vi "SMOOTHIE MAIN.vi"() -> ()   [LabVIEW 2016]
uses:
  PROCESSES.ctl
  <vilib>/Instr/_visa.llb/VISA Open Access Mode.ctl
panel:
  out "elements":T1[](array[typedef])
  out "CONNECTED":bool
  in  "ENABLE XYZ":bool
  out "GOTO STRING":string
  in  "ABS":bool
  in  "GOTO POSITION":T2 {"Z" format="%_4g"; "Y" min=-0.019999999552965164 max=0.019999999552965164 step=9.999999747378752e-05 format="%_5g"; "X" format="%_5g"}
  out "APOS":string
  in  "Stop Button":bool
  out "LIMITS":string
  in  "LIMITS":bool
  out "SMOOTHIE VISA":refnum<visa-resource-name>
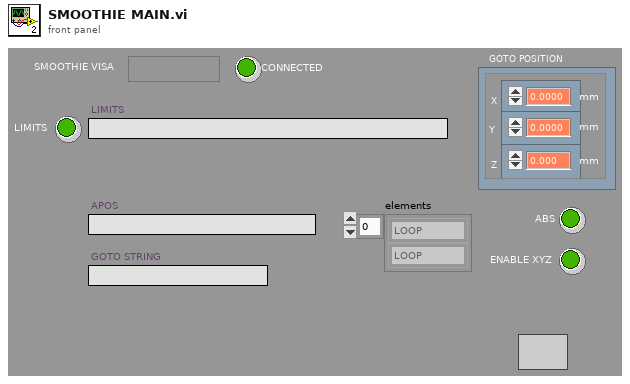
[diagram p1: front panel]
types:
  T1 = typedef "PROCESSES.ctl" = enum16{"LOOP", "LIMITS SETTINGS", "INITIALISE COMM", "CLOSE VISA COMM", "ACTUATOR POSITIONS", "GOTO POSITION (TOOL UP)", "ABSOLUTE or RELATIVE", "ENABLE STEPPER MOTORS"}
  T2 = cluster{"X":dbl[unit], "Y":dbl[unit], "Z":dbl[unit]}
  T3 = typedef "VISA Open Access Mode.ctl" = u32
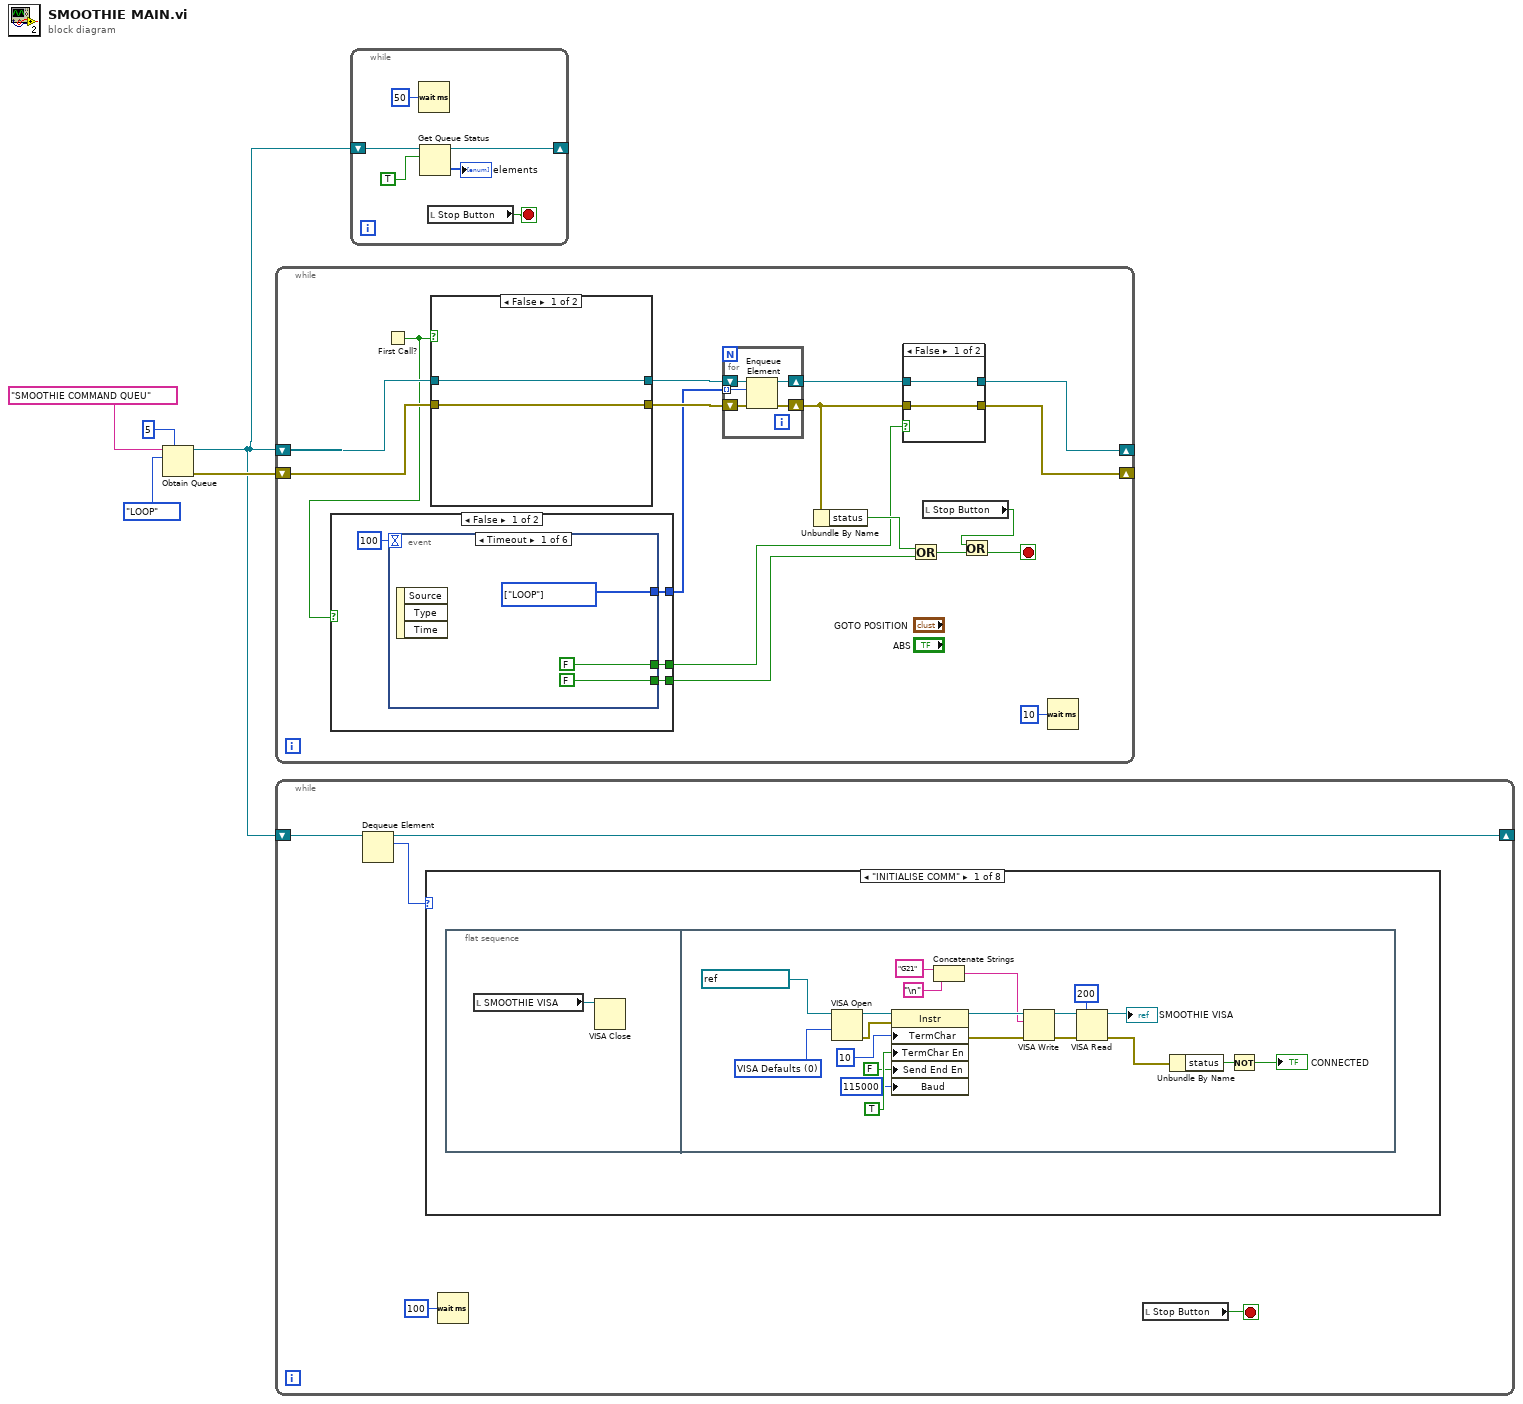
[diagram p0: block diagram]
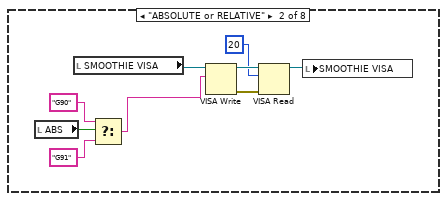
[diagram p2: hidden frame]
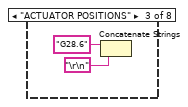
[diagram p3: hidden frame]
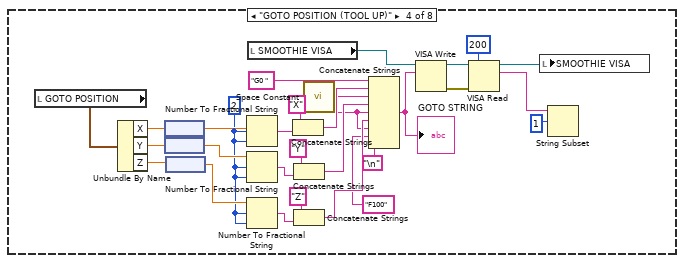
[diagram p4: hidden frame]
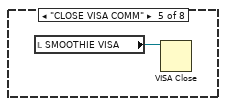
[diagram p5: hidden frame]
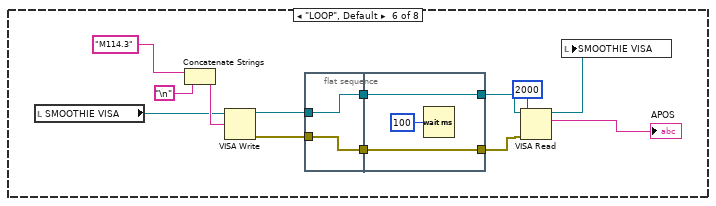
[diagram p6: hidden frame]
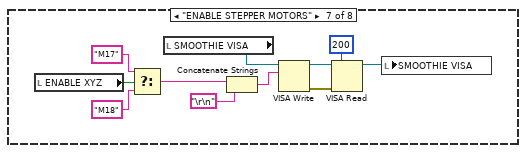
[diagram p7: hidden frame]
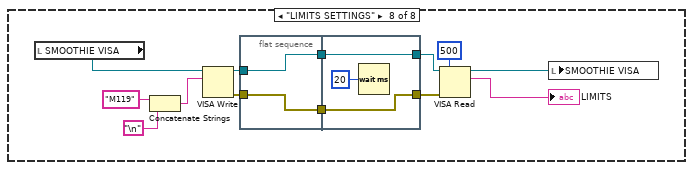
[diagram p8: hidden frame]
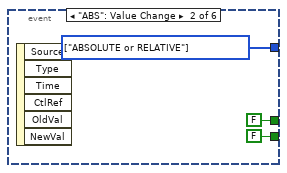
[diagram p9: hidden frame]
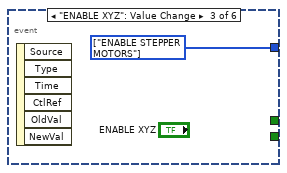
[diagram p10: hidden frame]
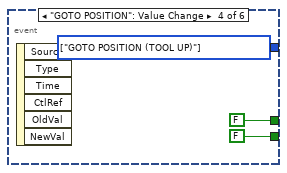
[diagram p11: hidden frame]
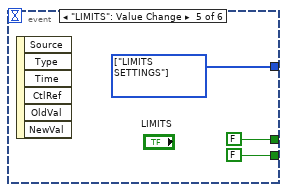
[diagram p12: hidden frame]
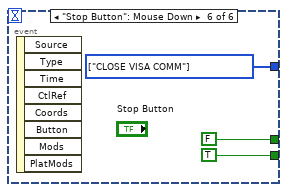
[diagram p13: hidden frame]
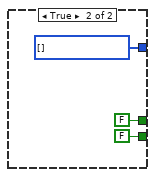
[diagram p14: hidden frame]
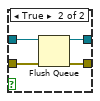
[diagram p15: hidden frame]
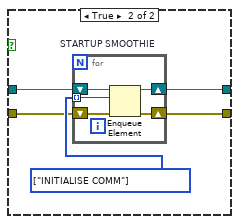
[diagram p16: hidden frame]
diagram:
  n1 = Obtain Queue(max queue size (-1, unlimited)=5, name (unnamed)="SMOOTHIE COMMAND QUEU", element data type=PROCESSES."LOOP") -> (queue out=w1:refnum<queue>, error out=w4:errorcluster)  [unwired: 2 in, 1 out]
  n2 = while {
    shift-right: [w11] -> _
    shift-left: w1 -> [w22]
    shift-right: [w10] -> _
    shift-left: w4 -> [w21]
    stop <- w9 stop-if-true
    n3 = First Call?() -> (First Call?: T/F=w12:bool)
    n4 = case shown="False" w12 {
      tunnel: [w25 w45] -> w18
      tunnel: [w24 FALSE] -> w16
      tunnel: [w23 FALSE] -> w14
      frame False {
        n5 = event shown="[0] Timeout" {
          selector: _ -> [_ _ _ _ _ _]
          dyn-events: _ -> [_ _ _ _ _ _]
          timeout: 100 -> [_ _ _ _ _ _]
          tunnel: [w29 w32 w33 w36 w39 w40] -> w25
          tunnel: [FALSE FALSE _ FALSE FALSE FALSE] -> w23
          tunnel: [FALSE FALSE _ FALSE FALSE TRUE] -> w24
          event Timeout {
            w29 = T1[] [enum."LOOP"] items=["LOOP", "LIMITS SETTINGS", "INITIALISE COMM", "CLOSE VISA COMM", "ACTUATOR POSITIONS", "GOTO POSITION (TOOL UP)", "ABSOLUTE or RELATIVE", "ENABLE STEPPER MOTORS"]
            n6 = event-data() -> ()  [unwired: 1 in, 3 out]
          }
          event "ABS": Value Change {
            w32 = T1[] [enum."ABSOLUTE or RELATIVE"] items=["LOOP", "LIMITS SETTINGS", "INITIALISE COMM", "CLOSE VISA COMM", "ACTUATOR POSITIONS", "GOTO POSITION (TOOL UP)", "ABSOLUTE or RELATIVE", "ENABLE STEPPER MOTORS"]
            n7 = event-data() -> ()  [unwired: 1 in, 6 out]
          }
          event "ENABLE XYZ": Value Change {
            w33 = T1[] [enum."ENABLE STEPPER MOTORS"] items=["LOOP", "LIMITS SETTINGS", "INITIALISE COMM", "CLOSE VISA COMM", "ACTUATOR POSITIONS", "GOTO POSITION (TOOL UP)", "ABSOLUTE or RELATIVE", "ENABLE STEPPER MOTORS"]
            n8 = event-data() -> ()  [unwired: 1 in, 6 out]
          }
          event "GOTO POSITION": Value Change {
            w36 = T1[] [enum."GOTO POSITION (TOOL UP)"] items=["LOOP", "LIMITS SETTINGS", "INITIALISE COMM", "CLOSE VISA COMM", "ACTUATOR POSITIONS", "GOTO POSITION (TOOL UP)", "ABSOLUTE or RELATIVE", "ENABLE STEPPER MOTORS"]
            n9 = event-data() -> ()  [unwired: 1 in, 6 out]
          }
          event "LIMITS": Value Change {
            w39 = T1[] [enum."LIMITS SETTINGS"] items=["LOOP", "LIMITS SETTINGS", "INITIALISE COMM", "CLOSE VISA COMM", "ACTUATOR POSITIONS", "GOTO POSITION (TOOL UP)", "ABSOLUTE or RELATIVE", "ENABLE STEPPER MOTORS"]
            n10 = event-data() -> ()  [unwired: 1 in, 6 out]
          }
          event "Stop Button": Mouse Down {
            w40 = T1[] [enum."CLOSE VISA COMM"] items=["LOOP", "LIMITS SETTINGS", "INITIALISE COMM", "CLOSE VISA COMM", "ACTUATOR POSITIONS", "GOTO POSITION (TOOL UP)", "ABSOLUTE or RELATIVE", "ENABLE STEPPER MOTORS"]
            n11 = event-data() -> ()  [unwired: 1 in, 8 out]
          }
        }
      }
      frame True {
        w45 = T1[] [] items=["LOOP", "LIMITS SETTINGS", "INITIALISE COMM", "CLOSE VISA COMM", "ACTUATOR POSITIONS", "GOTO POSITION (TOOL UP)", "ABSOLUTE or RELATIVE", "ENABLE STEPPER MOTORS"]
      }
    }
    n12 = case shown="False" w12 {
      tunnel: w22 -> [w58 w63]
      tunnel: w21 -> [w57 w61]
      tunnel: [w58 w60] -> w20
      tunnel: [w57 w59] -> w19
      frame False {
      }
      frame True {
        w62 = T1[] [enum."INITIALISE COMM"] items=["LOOP", "LIMITS SETTINGS", "INITIALISE COMM", "CLOSE VISA COMM", "ACTUATOR POSITIONS", "GOTO POSITION (TOOL UP)", "ABSOLUTE or RELATIVE", "ENABLE STEPPER MOTORS"]  # STARTUP SMOOTHIE
        n13 = for {
          tunnel: w62 -> [w67] mode=indexing
          shift-right: [w65] -> w59
          shift-left: w61 -> [w66]
          shift-right: [w64] -> w60
          shift-left: w63 -> [w68]
          n14 = Enqueue Element(queue=w68, element=w67, error in (no error)=w66) -> (queue out=w64:refnum<queue>, error out=w65:errorcluster)  [unwired: 1 in, 1 out]
        }
      }
    }
    n15 = for {
      tunnel: w18 -> [w55] mode=indexing
      shift-right: [w53] -> w13
      shift-left: w19 -> [w54]
      shift-right: [w52] -> w15
      shift-left: w20 -> [w56]
      n16 = Enqueue Element(queue=w56, element=w55, error in (no error)=w54) -> (queue out=w52:refnum<queue>, error out=w53:errorcluster)  [unwired: 1 in, 1 out]
    }
    n17 = Unbundle By Name(w13) -> ("status"=w17:bool)
    n18 = case shown="False" w14 {
      tunnel: w15 -> [w47 w51]
      tunnel: w13 -> [w46 w50]
      tunnel: [w47 w49] -> w11
      tunnel: [w46 w48] -> w10
      frame False {
      }
      frame True {
        n19 = Flush Queue(queue=w51, error in (no error)=w50) -> (queue out=w49:refnum<queue>, error out=w48:errorcluster)  [unwired: 1 out]
      }
    }
    n20 = Or(x=w17, y=w16) -> (x .or. y?=w8:bool)
    n21 = local read "Stop Button"() -> (w7:bool)
    n22 = Or(x=w7, y=w8) -> (x .or. y?=w9:bool)
    n23 = Wait (ms)(milliseconds to wait=u32 10) -> ()  [unwired: 1 out]
  }
  n24 = while {
    shift-right: [w71] -> _
    shift-left: w1 -> [w73]
    stop <- w70 stop-if-true
    n25 = Dequeue Element(queue=w73) -> (queue out=w71:refnum<queue>, element=w72:T1)  [unwired: 2 in, 2 out]
    n26 = case shown="\"INITIALISE COMM\"" w72 {
      frame "INITIALISE COMM" {
        n27 = flat-sequence {
          frame #0 {
            n28 = local read "SMOOTHIE VISA"() -> (w74:refnum<visa-resource-name>)
            n29 = VISA Close(VISA resource name=w74) -> ()  [unwired: 1 in, 1 out]
          }
          frame #1 {
            w88 = T3 0 items=["VISA Defaults"=0, "Exclusive Lock"=1, "Load Configured Settings"=4] ("Access Mode")
            n30 = VISA Open(access mode=w88, VISA resource name=refnum<visa-resource-name> "SMOOTHIE") -> (VISA resource name=w90:refnum<visa-resource-name>, error out=w89:errorcluster)  [unwired: 3 in]
            n31 = property class="Instr"(reference=w90, error in=w89, "TermChar"=u8 10 ("Message Based Settings:Termination Character"), "TermChar En"=TRUE ("Message Based Settings:Termination Character Enable"), "Send End En"=FALSE ("Message Based Settings:Send End Enable"), "Baud"=u32 115000 ("Serial Settings:Baud Rate")) -> (reference out=w87:refnum<visa-resource-name>, error out=w85:errorcluster)
            n32 = Concatenate Strings("G21" ("write buffer"), "\n") -> (w75:string)
            n33 = VISA Write(VISA resource name=w87, write buffer=w75, error in (no error)=w85) -> (VISA resource name out=w86:refnum<visa-resource-name>, error out=w84:errorcluster)  [unwired: 1 out]
            n34 = VISA Read(VISA resource name=w86, byte count=u32 200, error in (no error)=w84) -> (VISA resource name out=→"SMOOTHIE VISA":refnum<visa-resource-name>, error out=w78:errorcluster)  [unwired: 2 out]
            n35 = Unbundle By Name(w78) -> ("status"=w83:bool)
            n36 = Not(x=w83) -> (.not. x?=→"CONNECTED":bool)
          }
        }
      }
      frame "ABSOLUTE or RELATIVE" {
        n37 = local read "ABS"() -> (w100:bool)
        n38 = local read "SMOOTHIE VISA"() -> (w102:refnum<visa-resource-name>)
        n39 = Select(t="G90" ("write buffer"), s=w100, f="G91" ("write buffer")) -> (s? t:f=w95:string)
        n40 = VISA Write(VISA resource name=w102, write buffer=w95) -> (VISA resource name out=w101:refnum<visa-resource-name>, error out=w103:errorcluster)  [unwired: 1 in, 1 out]
        n41 = VISA Read(VISA resource name=w101, byte count=u32 20, error in (no error)=w103) -> (VISA resource name out=w97:refnum<visa-resource-name>)  [unwired: 3 out]
        n42 = local write "SMOOTHIE VISA"(w97) -> ()
      }
      frame "ACTUATOR POSITIONS" {
        n43 = Concatenate Strings("G28.6" ("write buffer"), "\r\n") -> ()  [unwired: 1 out]
      }
      frame "GOTO POSITION (TOOL UP)" {
        w111 = i16 2 ("width (-)")
        n44 = local read "GOTO POSITION"() -> (w134:T2)
        n45 = Unbundle By Name(w134) -> ("X"=w125:dbl[unit], "Y"=w124:dbl[unit], "Z"=w113:dbl[unit])
        n46 = node(w125) -> (w123:dbl)
        n47 = node(w124) -> (w122:dbl)
        n48 = node(w113) -> (w112:dbl)
        n49 = Number To Fractional String(number=w123, width (-)=w111, precision (6)=w111) -> (F-format string=w120:string)  [unwired: 1 in]
        n50 = Number To Fractional String(number=w122, width (-)=w111, precision (6)=w111) -> (F-format string=w117:string)  [unwired: 1 in]
        n51 = Number To Fractional String(number=w112, width (-)=w111, precision (6)=w111) -> (F-format string=w114:string)  [unwired: 1 in]
        n52 = local read "SMOOTHIE VISA"() -> (w126:refnum<visa-resource-name>)
        n53 = Concatenate Strings("X" ("string"), w120) -> (w119:string)
        n54 = Concatenate Strings("Y" ("string"), w117) -> (w115:string)
        n55 = Concatenate Strings("Z" ("string"), w114) -> (w109:string)
        n56 = call <vilib>:"Space Constant.vi"() -> ("String"=w108:string)
        n57 = Concatenate Strings("G0 " ("write buffer"), w119, w108, w115, w108, w109, w108, "F100", "\n") -> (w130:string)
        "GOTO STRING" <- w130
        n58 = VISA Write(VISA resource name=w126, write buffer=w130) -> (VISA resource name out=w132:refnum<visa-resource-name>, error out=w129:errorcluster)  [unwired: 1 in, 1 out]
        n59 = VISA Read(VISA resource name=w132, byte count=u32 200, error in (no error)=w129) -> (VISA resource name out=w121:refnum<visa-resource-name>, read buffer=w128:string)  [unwired: 2 out]
        n60 = local write "SMOOTHIE VISA"(w121) -> ()
        n61 = String Subset(string=w128, offset (0)=1) -> ()  [unwired: 1 in, 1 out]
      }
      frame "CLOSE VISA COMM" {
        n62 = local read "SMOOTHIE VISA"() -> (w135:refnum<visa-resource-name>)
        n63 = VISA Close(VISA resource name=w135) -> ()  [unwired: 1 in, 1 out]
      }
      frame "LOOP", Default {
        n64 = local read "SMOOTHIE VISA"() -> (w143:refnum<visa-resource-name>)
        n65 = Concatenate Strings("M114.3" ("write buffer"), "\n") -> (w145:string)
        n66 = VISA Write(VISA resource name=w143, write buffer=w145) -> (VISA resource name out=w142:refnum<visa-resource-name>, error out=w141:errorcluster)  [unwired: 1 in, 1 out]
        n67 = flat-sequence {
          tunnel: w142 -> [w150]
          tunnel: w141 -> [w149]
          tunnel: [w150] -> w139
          tunnel: [w149] -> w137
          tunnel: [w152] -> w140
          tunnel: w139 -> [w152]
          tunnel: [w151] -> w138
          tunnel: w137 -> [w151]
          frame #0 {
          }
          frame #1 {
            n68 = Wait (ms)(milliseconds to wait=u32 100) -> ()  [unwired: 1 out]
          }
        }
        n69 = VISA Read(VISA resource name=w140, byte count=u32 2000, error in (no error)=w138) -> (VISA resource name out=w144:refnum<visa-resource-name>, read buffer=→"APOS":string)  [unwired: 2 out]
        n70 = local write "SMOOTHIE VISA"(w144) -> ()
      }
      frame "ENABLE STEPPER MOTORS" {
        n71 = local read "ENABLE XYZ"() -> (w158:bool)
        n72 = Select(t="M17" ("write buffer"), s=w158, f="M18" ("write buffer")) -> (s? t:f=w155:string)
        n73 = local read "SMOOTHIE VISA"() -> (w159:refnum<visa-resource-name>)
        n74 = Concatenate Strings(w155, "\r\n") -> (w161:string)
        n75 = VISA Write(VISA resource name=w159, write buffer=w161) -> (VISA resource name out=w163:refnum<visa-resource-name>, error out=w160:errorcluster)  [unwired: 1 in, 1 out]
        n76 = VISA Read(VISA resource name=w163, byte count=u32 200, error in (no error)=w160) -> (VISA resource name out=w154:refnum<visa-resource-name>)  [unwired: 3 out]
        n77 = local write "SMOOTHIE VISA"(w154) -> ()
      }
      frame "LIMITS SETTINGS" {
        n78 = local read "SMOOTHIE VISA"() -> (w173:refnum<visa-resource-name>)
        n79 = Concatenate Strings("M119" ("write buffer"), "\n") -> (w172:string)
        n80 = VISA Write(VISA resource name=w173, write buffer=w172) -> (VISA resource name out=w168:refnum<visa-resource-name>, error out=w165:errorcluster)  [unwired: 1 in, 1 out]
        n81 = flat-sequence {
          tunnel: [w179] -> w169
          tunnel: w168 -> [w179]
          tunnel: [w178] -> w166
          tunnel: w165 -> [w178]
          tunnel: [w182] -> w170
          tunnel: w169 -> [w182]
          tunnel: [w181] -> w167
          tunnel: w166 -> [w181]
          frame #0 {
          }
          frame #1 {
            n82 = Wait (ms)(milliseconds to wait=u32 20) -> ()  [unwired: 1 out]
          }
        }
        n83 = VISA Read(VISA resource name=w170, byte count=u32 500, error in (no error)=w167) -> (VISA resource name out=w175:refnum<visa-resource-name>, read buffer=→"LIMITS":string)  [unwired: 2 out]
        n84 = local write "SMOOTHIE VISA"(w175) -> ()
      }
    }
    n85 = Wait (ms)(milliseconds to wait=u32 100) -> ()  [unwired: 1 out]
    n86 = local read "Stop Button"() -> (w70:bool)
  }
  n87 = while {
    shift-right: [w186] -> _
    shift-left: w1 -> [w187]
    stop <- w185 stop-if-true
    n88 = Wait (ms)(milliseconds to wait=u32 50) -> ()  [unwired: 1 out]
    n89 = Get Queue Status(queue=w187, return elements? (F)=TRUE) -> (queue out=w186:refnum<queue>, elements=→"elements":T1[])  [unwired: 1 in, 6 out]
    n90 = local read "Stop Button"() -> (w185:bool)
  }
